vi "User - Delete.vi"(8 "error in (no error)":errorcluster, 10 "User Pointer(1-299)":i32=1, 11 "VISA resource name":refnum<visa-resource-name>) -> (0 "error out":errorcluster, 3 "VISA resource name out":refnum<visa-resource-name>)   [LabVIEW 2014, in "eec EST 300.lvlib"]
doc: "Delete user"
uses:
  <instrlib>/eec EST 300/eec EST 300.lvlib
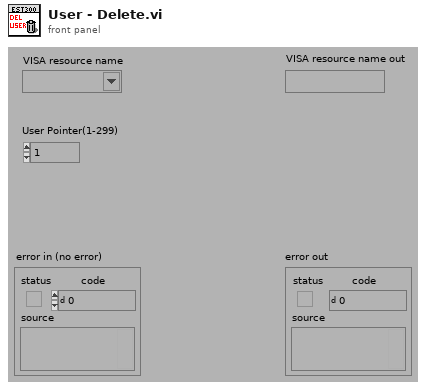
[diagram p1: front panel]
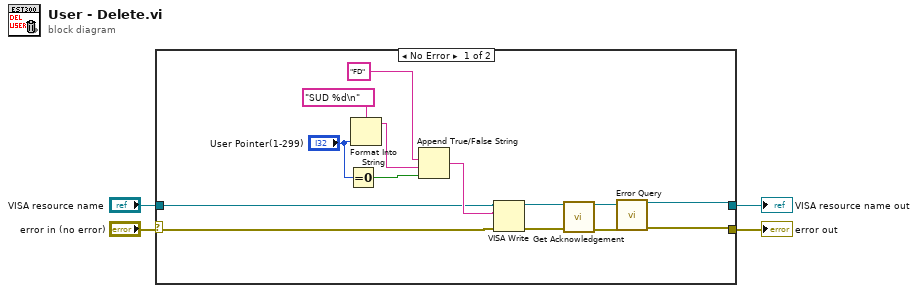
[diagram p0: block diagram]
diagram:
  n1 = case shown="No Error" "error in (no error)" {
    selector: "error in (no error)" -> [w9 w19]
    tunnel: "VISA resource name" -> [w7 w20]
    tunnel: [w5 w20] -> w3
    tunnel: [w6 w19] -> w2
    frame No Error {
      n2 = Equal To 0?(x="User Pointer(1-299)") -> (x = 0?=w16:bool)
      n3 = Format Into String(format string="SUD %d\n" ("\"False\" Command"), "User Pointer(1-299)") -> (resulting string=w15:string)  [unwired: 2 in, 1 out]
      n4 = Append True/False String(1:w16, 2:w15, 3:"FD" ("f")) -> (0:w8:string)  [unwired: 1 in]
      n5 = VISA Write(VISA resource name=w7, write buffer=w8, error in (no error)=w9) -> (VISA resource name out=w11:refnum<visa-resource-name>, error out=w10:errorcluster)  [unwired: 1 out]
      n6 = call <instrlib>:"Get Acknowledgement.vi"("VISA resource name"=w11, "error in (no error)"=w10) -> ("VISA resource name out"=w13:refnum<visa-resource-name>, "error out"=w12:errorcluster)  [unwired: 12 in]
      n7 = call <instrlib>:"Error Query.vi"("VISA resource name"=w13, "error in (no error)"=w12) -> ("VISA resource name out"=w5:refnum<visa-resource-name>, "error out"=w6:errorcluster)  [unwired: 10 in, 2 out]
    }
    frame Error {
    }
  }
  "error out" <- w2
  "VISA resource name out" <- w3
